vi "Create and Show Form.vi"() -> ()   [LabVIEW 2012, in "Form.lvlib"]
uses:
  Form.lvlib
  System.Windows.Forms
  System.Drawing
panel:
  in  "停止":bool
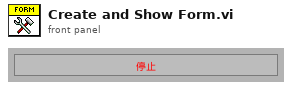
[diagram p1: front panel]
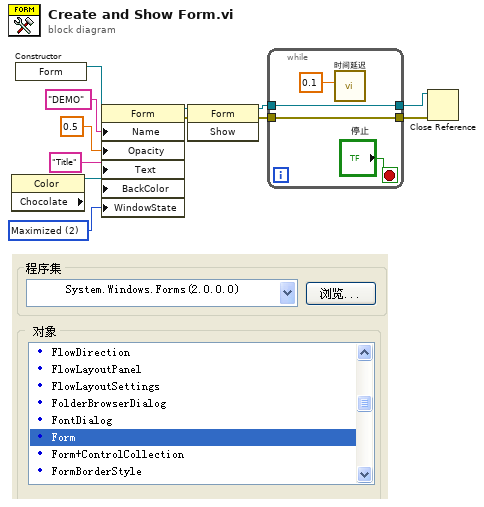
[diagram p0: block diagram]
diagram:
  w1 = 2 items=["Normal", "Minimized", "Maximized"] ("WindowState")
  n1 = property class="Color" props=["Chocolate"]() -> (reference out=w2:refnum<k24>)  [unwired: 2 in, 2 out]
  n2 = constructor class="Form"() -> (reference out=w12:refnum<k24>)  [unwired: 3 in, 2 out]
  n3 = property class="Form"(reference=w12, "Name"="DEMO", "Opacity"=0.5, "Text"="Title", "BackColor"=w2, "WindowState"=w1) -> (reference out=w10:refnum<k24>, error out=w9:errorcluster)  [unwired: 1 in]
  n4 = invoke class="Form" method="Show"(reference=w10, error in=w9) -> (reference out=w8:refnum<k24>, error out=w7:errorcluster)  [unwired: 1 in, 1 out]
  n5 = while {
    tunnel: w8 -> [w14]
    tunnel: w7 -> [w13]
    tunnel: [w14] -> w6
    tunnel: [w13] -> w5
    stop <- "停止" stop-if-true
    n6 = call "时间延迟"("Delay Time (s)"=0.1) -> ()  [unwired: 10 in, 1 out]
  }
  n7 = Close Reference(reference=w6, error in (no error)=w5) -> ()  [unwired: 1 out]
